vi "time_series_to_js.vi"(5 "names":string[](array[string]), 6 "time array name":string, 7 "Array":dbl[][](array[numeric]), 8 "time array":timestamp[](array[timestamp]), 10 "file path (use dialog)":path) -> (0 "web page write":errorcluster)   [LabVIEW 2013]
doc: "Save some time-series data to a .js file."
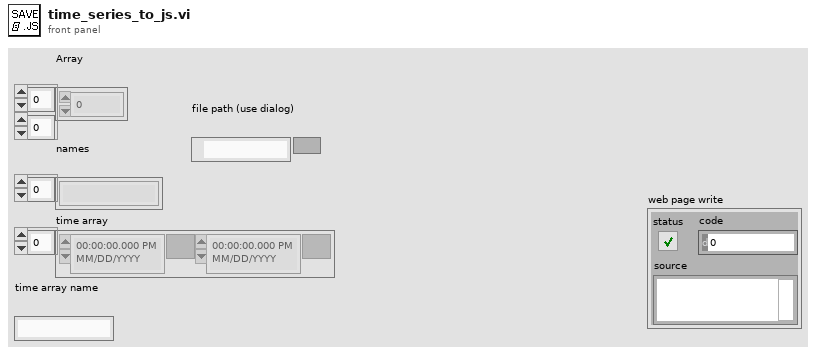
[diagram p1: front panel]
types:
  T1 = enum16{"open", "replace", "create", "open or create", "replace or create", "replace or create with confirmation"}
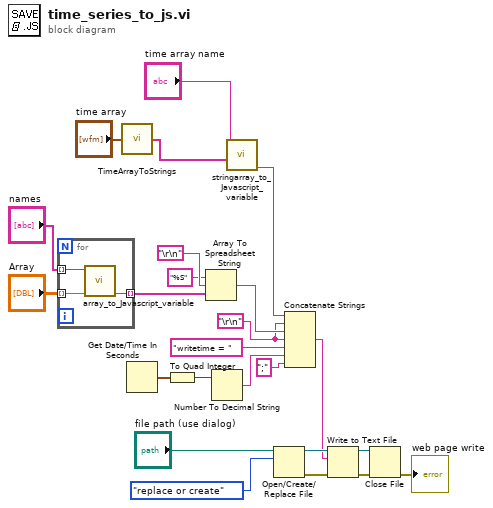
[diagram p0: block diagram]
diagram:
  w3 = "\r\n"
  n1 = for {
    tunnel: "Array" -> [w27] mode=indexing
    tunnel: "names" -> [w26] mode=indexing
    tunnel: [w25] -> w13 mode=indexing
    n2 = call "array_to_Javascript_variable.vi"("array"=w27, "variable_name"=w26) -> ("variable_string"=w25:string)  [unwired: 8 in]
  }
  n3 = call "TimeArrayToStrings.vi"("Array"="time array") -> ("time strings"=w4:string[])  [unwired: 2 in]
  n4 = Get Date/Time In Seconds() -> (seconds since 1Jan1904=w12:timestamp)
  n5 = To Quad Integer(1:w12) -> (0:w11:i64)
  n6 = Array To Spreadsheet String(delimiter (Tab)="\r\n", array=w13, 3:"%S" ("format string")) -> (spreadsheet string=w6:string)
  n7 = Number To Decimal String(number=w11) -> (decimal integer string=w9:string)  [unwired: 1 in]
  n8 = call "stringarray_to_Javascript_variable.vi"("Array"=w4, "variable_name"="time array name") -> ("variable_string"=w2:string)  [unwired: 8 in]
  n9 = Open/Create/Replace File(file path (use dialog)="file path (use dialog)", operation (0:open)=T1."replace or create") -> (refnum out=w19:refnum<file>, error out=w16:errorcluster)  [unwired: 4 in, 1 out]
  n10 = Concatenate Strings(w2, w3, w6, w3, "writetime = " ("string"), w9, ";" ("string")) -> (w7:string)
  n11 = Write to Text File(file (use dialog)=w19, text=w7, error in=w16) -> (refnum out=w18:refnum<file>, error out=w17:errorcluster)  [unwired: 1 in, 1 out]
  n12 = Close File(refnum=w18, error in=w17) -> (error out=→"web page write":errorcluster)  [unwired: 1 out]
